vi "Hastie_10_2.vi"(8 "error in (no error)":errorcluster caption="entrée d'erreur (pas d'erreur)", 11 "make_hastie_10_2":T2={"n_samples"=12000, "random_state"=-1, "Returns"="X"} {"random_state" min=-1; "n_samples" min=1}) -> (0 "error out":errorcluster, 3 "Data":T1)   [LabVIEW 2020]
doc: "Generates data for binary classification used in Hastie et al. 2009, Example 10.2.\n\nThe ten features are standard independent Gaussian and the target y is defined by:\n\ny[i] = 1 if np.sum(X[i] ** 2) > 9.34 else -1\n\n\n\nParameters :\n\n- n_samples : int, optional (default=12000)\nThe number of samples.\n\n- random_state : int, RandomState instance, default=None=-1\nDetermines random number generation for dataset creation. Pass an int for reproducible output across multiple function calls. See Glossary.\n\nReturns :\n\n- X : array of shape [n_samples, 10]\nThe input samples.\n\n- y : array of shape [n_samples]\nThe output values."
uses:
  Hastie_10_2.lvclass
panel:
  out "Hastie_10_2.lvclass":refnum<class "Hastie_10_2.lvclass">
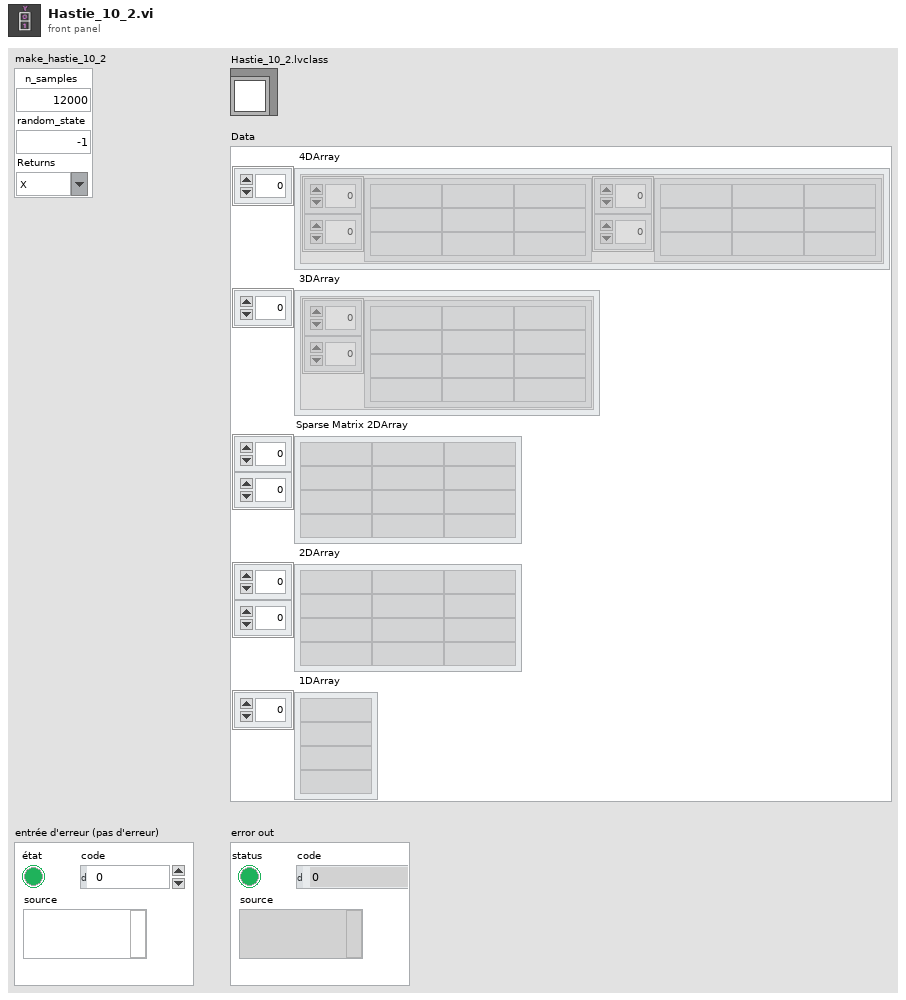
[diagram p1: front panel]
types:
  T1 = cluster{" 4DArray":cluster{"1":string[][], "2":string[][]}[], " 3DArray":cluster{"Tableau":string[][]}[], "Sparse Matrix 2DArray":string[][], " 2DArray":string[][], " 1DArray":string[]}
  T2 = cluster{"n_samples":u32, "random_state":i32, "Returns":string}
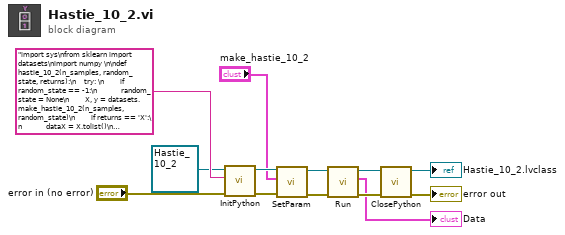
[diagram p0: block diagram]
diagram:
  n1 = call-dynamic "InitPython.vi"("error in (no error)"="error in (no error)", "Python Instruction"="import sys\nfrom sklearn import datasets\nimport numpy \n\ndef hastie_10_2(n_samples, random_state, returns):\n    try: \n        if random_state == -1:\n            random_state = None\n        X, y = datasets.make_hastie_10_2(n_samples, random_state)\n        if returns == 'X':\n            dataX = X.tolist()\n            return str(dataX)\n        else :\n            datay = y.tolist()\n            return str(datay)\n    except:\n        erreur = sys.exc_info()\n        typerr = u\"%s\" % (erreur[0])\n        typerr = typerr[typerr.find(\"'\")+1:typerr.rfind(\"'\")]\n        msgerr = u\"%s\" % (erreur[1])\n        message = str('/!\\\\ {0} : {1}'. format(typerr,msgerr))\n        return message", "Scikit-learn en entrée"=refnum<class "Hastie_10_2.lvclass"> refnum ("Hastie_10_2.lvclass")) -> ("error out"=w9:errorcluster, "Scikit-learn en sortie"=w10:refnum<class "Hastie_10_2.lvclass">)  [unwired: 7 in]
  n2 = call-dynamic "SetParam.vi"("error in (no error)"=w9, "make_hastie_10_2"="make_hastie_10_2", "Hastie_10_2.lvclass"=w10) -> ("error out"=w6:errorcluster, "Hastie_10_2.lvclass"=w7:refnum<class "Hastie_10_2.lvclass">)  [unwired: 7 in]
  n3 = call-dynamic "Run.vi"("error in (no error)"=w6, "Hastie_10_2.lvclass"=w7) -> ("error out"=w4:errorcluster, "Data"=→"Data":T1, "Hastie_10_2.lvclass"=w5:refnum<class "Hastie_10_2.lvclass">)  [unwired: 7 in]
  n4 = call-dynamic "ClosePython.vi"("error in (no error)"=w4, "Scikit-learn en entrée"=w5) -> ("error out"=→"error out":errorcluster, "Scikit-learn en sortie"=→"Hastie_10_2.lvclass":refnum<class "Hastie_10_2.lvclass">)  [unwired: 8 in]
